vi "Encapsulate Error.vi"(8 "error in (no error)":errorcluster, 9 "error size":T1=enum."512", 10 "address":u64 format="%016x") -> (0 "error out":errorcluster, 3 "Error Pointer out":refnum<class "Error Pointer.lvclass">)   [LabVIEW 2017, in "DSF Core.lvlib" / "Error Pointer.lvclass"]
uses:
  Error Pointer.lvclass
  C:/Program Files (x86)/National Instruments/LabVIEW 2017/vi.lib/NI/Memory Manager/Classes/Pointer/Pointer.lvclass
  Error Sizes.ctl
  Error Pointer.lvclass/Error Pointer.ctl
  <vilib>/NI/Memory Manager/Classes/Pointer/Pointer.lvclass/Pointer.ctl
  <vilib>/NI/Memory Manager/Classes/Pointer/Set Size.vi
  <vilib>/NI/Memory Manager/Classes/Pointer/Set Address.vi
  <vilib>/NI/Memory Manager/Classes/Pointer/Check Null Pointer.vi
  <vilib>/NI/Memory Manager/Classes/Pointer/Set Internal.vi
  <vilib>/NI/Memory Manager/Classes/Pointer/Errors.vi
  <vilib>/NI/Memory Manager/Classes/Pointer/Null Pointer.vi
  <vilib>/NI/Memory Manager/Classes/Pointer/Is Null.vi
  <vilib>/NI/Memory Manager/Classes/Pointer/Create Error.vi
  <vilib>/NI/Memory Manager/Classes/Pointer/Get Address.vi
  <vilib>/NI/Memory Manager/Constants/Constants.vi
  <vilib>/NI/Memory Manager/Constants/Library Name.vi
  <vilib>/NI/Memory Manager/Classes/Pointer/Pointer Error Info.vi
  <vilib>/NI/Memory Manager/Constants/Pointer Class Name.vi
  <vilib>/NI/Memory Manager/VIs/New Error Cluster.vi
  <vilib>/NI/Memory Manager/VIs/New Error Cluster (512B).vi
  <vilib>/NI/Memory Manager/VIs/Set Error Status.vi
  <vilib>/NI/Memory Manager/VIs/Set Error Code.vi
  <vilib>/NI/Memory Manager/VIs/Set Error Source.vi
  <vilib>/NI/Memory Manager/VIs/Write String to Source.vi
  <vilib>/NI/Memory Manager/Classes/Pointer/Pointer.lvclass
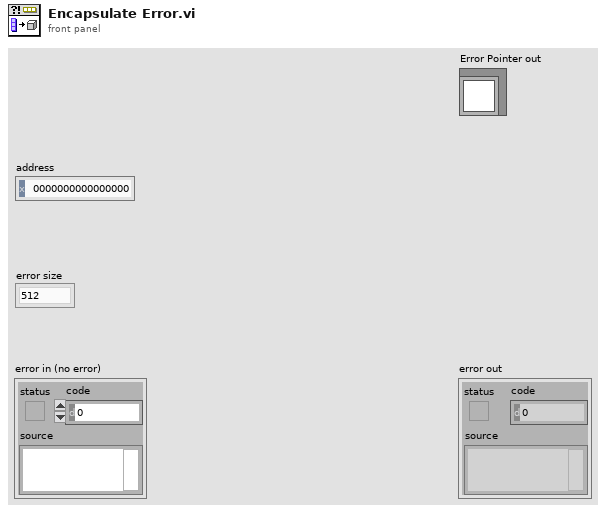
[diagram p1: front panel]
types:
  T1 = typedef "DSF Core.lvlib/Error Pointer.lvclass/Error Sizes.ctl" = enum8{"256", "512", "1024"}
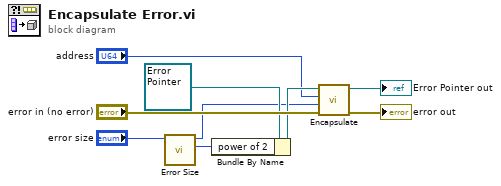
[diagram p0: block diagram]
diagram:
  n1 = call "Error Size.vi"("error size"="error size") -> ("power of 2"=w7:i16, "size"=w1:u64)  [unwired: 9 in]
  n2 = Bundle By Name(cluster=refnum<class "Error Pointer.lvclass"> refnum ("Error Pointer in"), "power of 2"=w7) -> (w4:refnum<class "Error Pointer.lvclass">)
  n3 = call <vilib>:"Encapsulate.vi"("error in (no error)"="error in (no error)", "size"=w1, "address"="address", "Pointer type"=w4) -> ("error out"=→"error out":errorcluster, "Pointer"=→"Error Pointer out":refnum<class "Error Pointer.lvclass">)  [unwired: 6 in]
